vi "EscapeString.vi"(0 "String":string, 11 "error in":errorcluster) -> (4 "Escaped String":string, 15 "error out":errorcluster)   [LabVIEW 2020, in "Redis.lvclass"]
doc: "Escapes the illegal characters of a string"
uses:
  Redis.lvclass
  Redis.lvclass/Redis.ctl
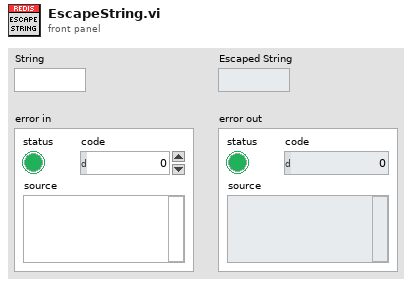
[diagram p1: front panel]
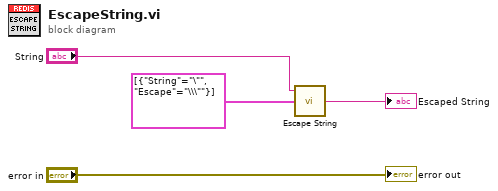
[diagram p0: block diagram]
diagram:
  n1 = call <vilib>:"Escape String.vi"("Escapes"=cluster{"String":string, "Escape":string}[] [{"String"="\"", "Escape"="\\\""}], "String in"="String") -> ("String out"=→"Escaped String":string)  [unwired: 1 in]
  "error out" <- "error in"
